vi "Begin.vi"() -> (0 "CameraDevRef 2":T1, 1 "CameraDevRef":T1)   [LabVIEW 2011]
doc: "Called before other user functions, this VI is expected to open initial I/O refnums, load in file data, and do all program initialization. Notice that the <B>error out</B> terminal is simply used for data flow. Wiring it to other structures or subVIs ensures that this VI runs first."
uses:
  <vilib>/Rock Robotics/WPI/Camera/WPI_CameraDevRef.ctl
  <vilib>/Rock Robotics/SystemInterfaces/DIO/FPGA_DIOPWMChannel.ctl
  <vilib>/Rock Robotics/WPI/Joystick/WPI_JoystickDeviceEnum.ctl
  <vilib>/Rock Robotics/SystemInterfaces/AI/FPGA_AIChannel.ctl
  <vilib>/Rock Robotics/SystemInterfaces/DIO/FPGA_DIORelayChannel.ctl
  <vilib>/Rock Robotics/SystemInterfaces/DIO/FPGA_DIOChannel.ctl
  <vilib>/Rock Robotics/SystemInterfaces/AI/FPGA_AIGyroChannel.ctl
  <vilib>/Rock Robotics/WPI/Relay/WPI_RelayDirection.ctl
  <vilib>/Rock Robotics/WPI/Encoder/WPI_EncoderType.ctl
  <vilib>/Rock Robotics/WPI/DriverStation/DriverStationLCD/WPI_DriverStationLCDLCDLine.ctl
  <vilib>/Rock Robotics/WPI/MotorControl/WPI_MotorControlOpen Victor.vi
  <vilib>/Rock Robotics/WPI/MotorControl/WPI_MotorControlOpen Jaguar.vi
  Robot Global Data.vi
  <vilib>/Utility/file.llb/Read From Spreadsheet File (DBL).vi
  <vilib>/Rock Robotics/WPI/Counter/WPI_CounterDigitalInputToDigitalSource.vi
  <vilib>/Rock Robotics/SystemInterfaces/Typedef/FPGA_TypedefDigitalModule.ctl
  <vilib>/Rock Robotics/SystemInterfaces/Typedef/FPGA_TypedefAnalogModule.ctl
panel:
  out "Path and file":string
  in  "Balls In Robot At Start":dbl=2.0
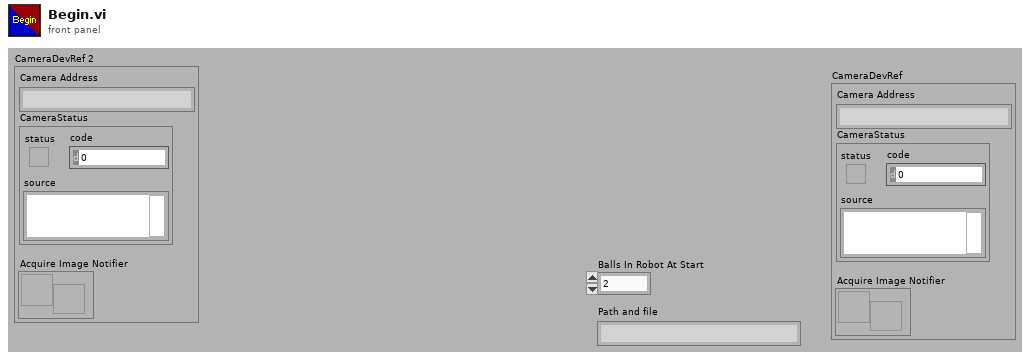
[diagram p1: front panel]
types:
  T1 = typedef "WPI_CameraDevRef.ctl" = cluster{"Camera Address":string, "CameraStatus":errorcluster, "Acquire Image Notifier":refnum<notifier>}
  T2 = typedef "WPI_DriverStationLCDLCDLine.ctl" = enum16{"Main - Line 1", "User - Line 2", "User - Line 3", "User - Line 4", "User - Line 5", "User - Line 6"}
  T3 = typedef "WPI_EncoderType.ctl" = enum16{"1x", "2x", "4x"}
  T4 = typedef "FPGA_DIOChannel.ctl" = enum8{"DIO 1", "DIO 2", "DIO 3", "DIO 4", "DIO 5", "DIO 6", "DIO 7", "DIO 8", "DIO 9", "DIO 10", "DIO 11", "DIO 12", "DIO 13", "DIO 14", "Invalid"}
  T5 = typedef "FPGA_DIORelayChannel.ctl" = enum8{"Relay 1", "Relay 2", "Relay 3", "Relay 4", "Relay 5", "Relay 6", "Relay 7", "Relay 8", "Invalid"}
  T6 = typedef "WPI_RelayDirection.ctl" = enum16{"Both directions", "Forward only", "Reverse only"}
  T7 = typedef "FPGA_AIGyroChannel.ctl" = enum8{"AI 1", "AI 2", "Invalid"}
  T8 = typedef "FPGA_DIOPWMChannel.ctl" = enum8{"PWM 1", "PWM 2", "PWM 3", "PWM 4", "PWM 5", "PWM 6", "PWM 7", "PWM 8", "PWM 9", "PWM 10", "Invalid"}
  T9 = typedef "FPGA_AIChannel.ctl" = enum8{"AI 1", "AI 2", "AI 3", "AI 4", "AI 5", "AI 6", "AI 7", "AI 8", "Invalid"}
  T10 = typedef "WPI_JoystickDeviceEnum.ctl" = enum16{"USB 1", "USB 2", "USB 3", "USB 4", "Kinect 1", "Kinect 2"}
  T11 = typedef "WPI_CameraImageSize.ctl" = enum16{"640x480", "320x240", "160x120"}
  T12 = cluster{"fps":i32, "compression":i32, "Image Size":T11}
  T13 = typedef "WPI_MotorControlDeviceRef.ctl" = cluster{"DeviceStatus":errorcluster, "Type":enum16{"PWM", "CAN"}, "PWM":cluster{"Digital Module":T14, "PWM Channel":T8, "DeadBand":T15}, "CAN":cluster{"Device Number":u8, "Control Mode":T16, "Semaphore":T17, "Max Vout":dbl}, "Invert":bool, "TransformRef":T18, "InvTransformRef":T18}
  T14 = typedef "FPGA_TypedefDigitalModule.ctl" = enum16{"Digital Module 1", "Digital Module 2"}
  T15 = typedef "WPI_PWMDeadband.ctl" = cluster{"Name":string, "maxPositivePwm":i32, "minPositivePwm":i32, "centerPwm":i32, "maxNegativePwm":i32, "minNegativePwm":i32, "angularRange":u16}
  T16 = typedef "WPI_CANJaguar_ControlMode.ctl" = enum8{"Percent VBus", "Current", "Speed", "Position", "Voltage"}
  T17 = typedef "Semaphore RefNum" = refnum<k1>
  T18 = typedef "WPI_PWMTransform_ConPane.ctl" = refnum<vi>
  T19 = typedef "WPI_ServoDeviceRef.ctl" = cluster{"DeviceStatus":errorcluster, "Digital Module":T14, "PWM Channel":T8, "DeadBand":T15}
  T20 = typedef "WPI_AnalogChannelDevRef.ctl" = cluster{"DevStatus":errorcluster, "Analog Module":T21, "Analog Channel":T9}
  T21 = typedef "FPGA_TypedefAnalogModule.ctl" = enum16{"Analog Module 1", "Analog Module 2"}
  T22 = typedef "WPI_CameraWhite Balance Values.ctl" = enum16{"Auto", "Fixed indoor", "Fixed outdoor 1", "Fixed outdoor 2", "Fixed fluorescent 1", "Fixed fluorescent 2", "Hold current"}
  T23 = typedef "WPI_JoystickDevRef.ctl" = cluster{"Device":T10}
  T24 = typedef "WPI_RelayDevRef.ctl" = cluster{"DevStatus":errorcluster, "Relay Channel":T5, "Digital Module":T14, "Relay Direction":T6}
  T25 = typedef "WPI_CameraExposure Values.ctl" = enum16{"Auto", "Flicker-free 50 Hz", "Flicker-free 60 Hz", "Hold current"}
  T26 = typedef "WPI_DigitalInputDevRef.ctl" = cluster{"DevStatus":errorcluster, "DIO Channel":T4, "Digital Module":T14}
  T27 = typedef "FPGA_CounterEncoderSourceConvertionLVSourceType.ctl" = cluster{"DevStatus":errorcluster, "AnalogTriggerMode?":bool, "DigitalMode":cluster{"Digital Module":T14, "DIO Channel":T28}, "AnalogTriggerMode":cluster{"AnalogTriggerIndex":T29, "OutputType":T30}}
  T28 = typedef "FPGA_DIODigitalSourceChannel.ctl" = enum8{"DIO 1", "DIO 2", "DIO 3", "DIO 4", "DIO 5", "DIO 6", "DIO 7", "DIO 8", "DIO 9", "DIO 10", "DIO 11", "DIO 12", "DIO 13", "DIO 14", "Disabled"}
  T29 = typedef "FPGA_AnalogTriggerIndex.ctl" = enum8{"Trig 0", "Trig 1", "Trig 2", "Trig 3", "Trig 4", "Trig 5", "Trig 6", "Trig 7", "Invalid"}
  T30 = typedef "FPGA_AnalogTriggerOutType.ctl" = enum16{"InWindow", "TriggerState", "Rising", "Falling"}
  T31 = typedef "WPI_EncoderDevRef.ctl" = cluster{"DevStatus":errorcluster, "EncoderIndex":T32, "CounterIndex":T33, "DistancePerCount":dbl, "Decoding Type":T3}
  T32 = typedef "FPGA_EncoderIdx.ctl" = enum8{"Enc 0", "Enc 1", "Enc 2", "Enc 3", "Invalid"}
  T33 = typedef "FPGA_CounterCtrSystemIndex.ctl" = enum8{"Ctr 0", "Ctr 1", "Ctr 2", "Ctr 3", "Ctr 4", "Ctr 5", "Ctr 6", "Ctr 7", "Invalid"}
  T34 = typedef "WPI_GyroDevRef.ctl" = cluster{"DevStatus":errorcluster, "Analog Module":T21, "Analog Channel":T9, "Offset":dbl, "Gain (VoltsPerDegree/Second)":dbl}
  T35 = typedef "WPI_UltrasonicDeviceRef.ctl" = cluster{"DevStatus":errorcluster, "Ping Digital Module":T14, "Echo Digital Module":T14, "Ping Channel":T4, "Echo Channel":T4, "CntIndex":T33}
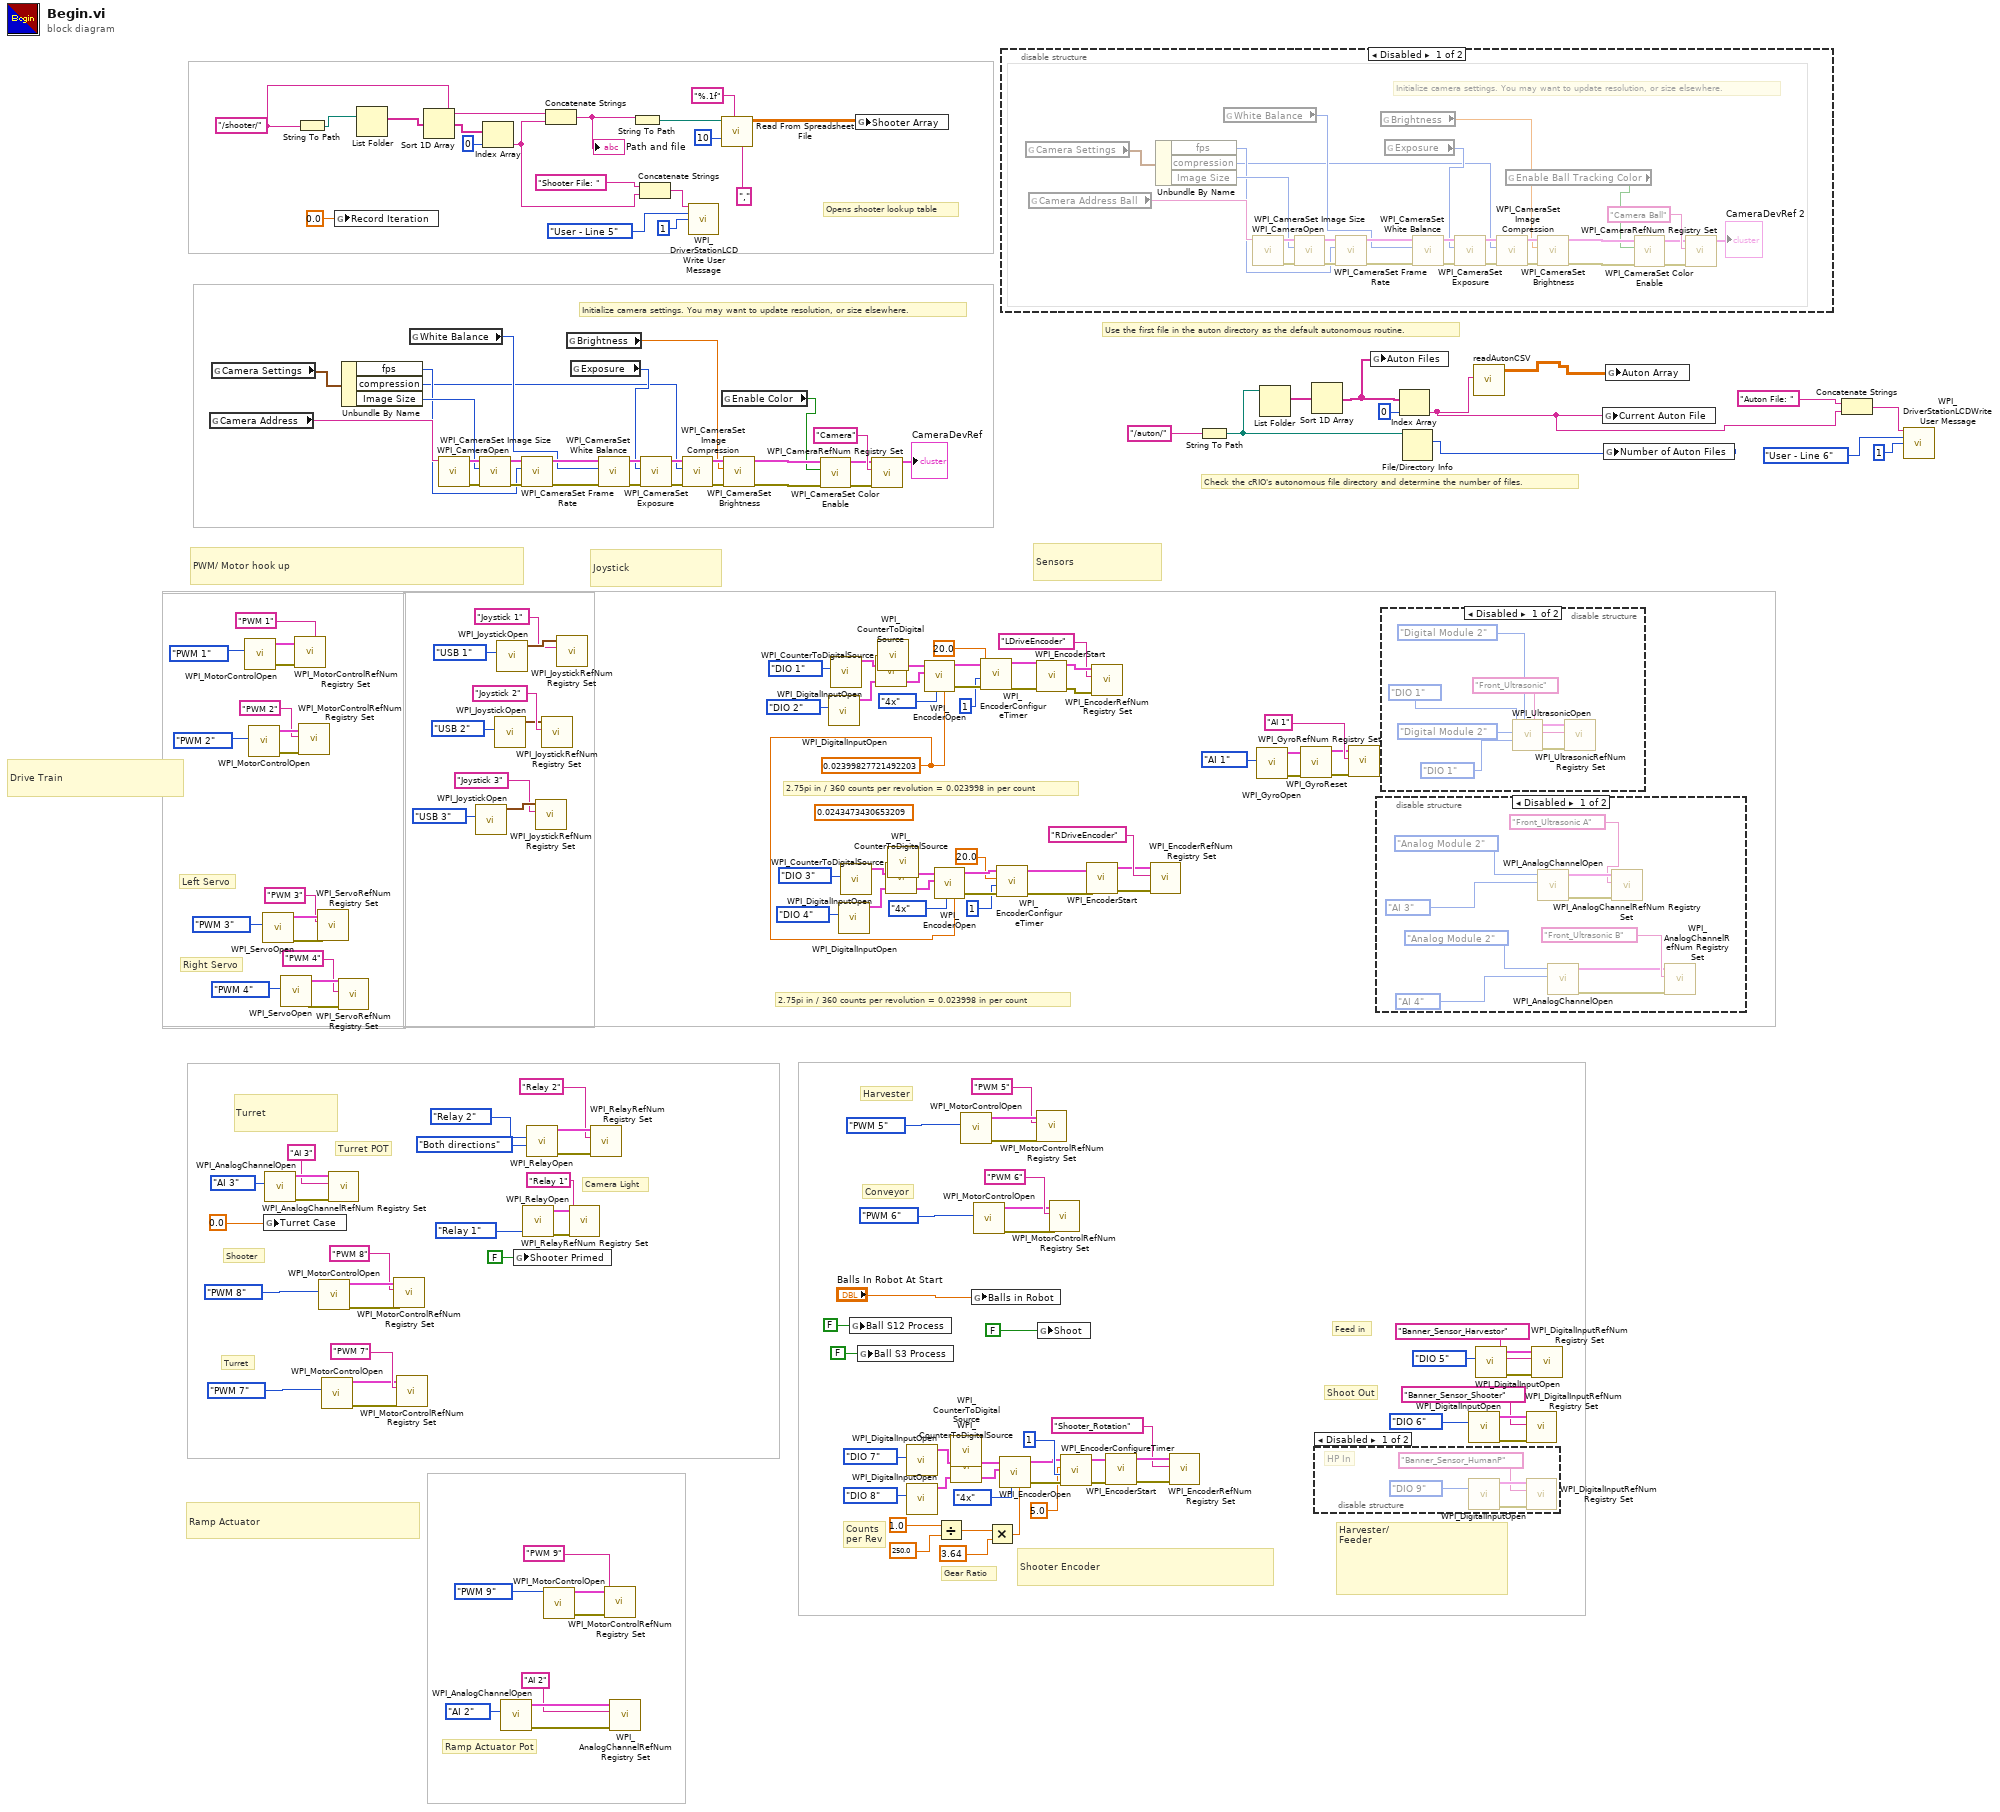
[diagram p0: block diagram]
diagram:
  (unwired) 0.0243473430653209 ("DistancePerCount")
  w32 = 0.02399827721492203 ("DistancePerCount")
  w80 = "/shooter/" ("string")
  # "Shooter Encoder"
  # "Counts\nper Rev"
  # "Gear Ratio"
  # "Check the cRIO's autonomous file directory and determine the number of files."
  # "Use the first file in the auton directory as the default autonomous routine."
  # "2.75pi in / 360 counts per revolution = 0.023998 in per count"
  # "2.75pi in / 360 counts per revolution = 0.023998 in per count"
  # "Opens shooter lookup table"
  # "Shoot Out"
  # "Feed in"
  # "Harvester"
  # "Conveyor"
  # "Shooter"
  # "Initialize camera settings. You may want to update resolution, or size elsewhere."
  # "Camera Light"
  # "Ramp Actuator Pot"
  # "Turret POT"
  # "Turret"
  # "Right Servo"
  # "Left Servo"
  # "Harvester/\nFeeder"
  # "Turret"
  # "Ramp Actuator"
  # "Drive Train"
  # "Sensors"
  # "Joystick"
  # "PWM/ Motor hook up"
  n1 = global read "Robot Global Data.vi" "Camera Address"() -> (w133:string)
  n2 = global read "Robot Global Data.vi" "Camera Settings"() -> (w132:T12)
  n3 = call-poly <vilib>:"WPI_MotorControlOpen.vi"("PWM Channel"=FPGA_DIOPWMChannel."PWM 1") -> ("error out"=w173:errorcluster, "MotorControlDeviceRef"=w175:T13)  [unwired: 9 in]
  n4 = call-poly <vilib>:"WPI_MotorControlOpen.vi"("PWM Channel"=FPGA_DIOPWMChannel."PWM 2") -> ("error out"=w171:errorcluster, "MotorControlDeviceRef"=w169:T13)  [unwired: 9 in]
  n5 = call <vilib>:"WPI_ServoOpen.vi"("PWM Channel"=FPGA_DIOPWMChannel."PWM 3") -> ("error out"=w186:errorcluster, "ServoDeviceRef"=w191:T19)  [unwired: 9 in]
  n6 = global write "Robot Global Data.vi" "Turret Case"(0.0 ("Return To Home Case")) -> ()
  n7 = call <vilib>:"WPI_AnalogChannelOpen.vi"("Analog Channel"=FPGA_AIChannel."AI 3") -> ("error out"=w162:errorcluster, "AIDeviceRef"=w163:T20)  [unwired: 9 in]
  n8 = call <vilib>:"WPI_ServoOpen.vi"("PWM Channel"=FPGA_DIOPWMChannel."PWM 4") -> ("error out"=w185:errorcluster, "ServoDeviceRef"=w189:T19)  [unwired: 9 in]
  n9 = call <vilib>:"WPI_MotorControlRefNum Registry Set.vi"("error in (no error)"=w173, "refnum name"="PWM 1", "MotorControlDevRef"=w175) -> ()  [unwired: 7 in, 2 out]
  n10 = String To Path(string=w80) -> (path=w89:path)
  n11 = call <vilib>:"WPI_MotorControlRefNum Registry Set.vi"("error in (no error)"=w171, "refnum name"="PWM 2", "MotorControlDevRef"=w169) -> ()  [unwired: 7 in, 2 out]
  n12 = call <vilib>:"WPI_ServoRefNum Registry Set.vi"("error in (no error)"=w186, "refnum name"="PWM 3", "ServoDeviceRef"=w191) -> ()  [unwired: 7 in, 2 out]
  n13 = call-poly <vilib>:"WPI_MotorControlOpen.vi"("PWM Channel"=FPGA_DIOPWMChannel."PWM 8") -> ("error out"=w116:errorcluster, "MotorControlDeviceRef"=w118:T13)  [unwired: 9 in]
  n14 = call-poly <vilib>:"WPI_MotorControlOpen.vi"("PWM Channel"=FPGA_DIOPWMChannel."PWM 7") -> ("error out"=w167:errorcluster, "MotorControlDeviceRef"=w165:T13)  [unwired: 9 in]
  n15 = call <vilib>:"WPI_AnalogChannelRefNum Registry Set.vi"("error in (no error)"=w162, "refnum name"="AI 3", "AIDeviceRef"=w163) -> ()  [unwired: 7 in, 2 out]
  n16 = global write "Robot Global Data.vi" "Record Iteration"(0.0 ("Record Iteration")) -> ()
  n17 = call <vilib>:"WPI_ServoRefNum Registry Set.vi"("error in (no error)"=w185, "refnum name"="PWM 4", "ServoDeviceRef"=w189) -> ()  [unwired: 7 in, 2 out]
  n18 = Unbundle By Name(w132) -> ("fps"=w130:i32, "compression"=w127:i32, "Image Size"=w131:T11)
  n19 = List Folder(path=w89) -> (filenames=w88:string[])  [unwired: 1 in, 5 out]
  n20 = call <vilib>:"WPI_MotorControlRefNum Registry Set.vi"("error in (no error)"=w116, "refnum name"="PWM 8", "MotorControlDevRef"=w118) -> ()  [unwired: 7 in, 2 out]
  n21 = call <vilib>:"WPI_MotorControlRefNum Registry Set.vi"("error in (no error)"=w167, "refnum name"="PWM 7", "MotorControlDevRef"=w165) -> ()  [unwired: 7 in, 2 out]
  n22 = global read "Robot Global Data.vi" "White Balance"() -> (w129:T22)
  n23 = Sort 1D Array(array=w88) -> (sorted array=w87:string[])
  n24 = call <vilib>:"WPI_CameraOpen.vi"("Camera Address"=w133) -> ("error out"=w139:errorcluster, "CameraDevRef"=w140:T1)  [unwired: 1 in, 8 out]
  n25 = call <vilib>:"WPI_JoystickOpen.vi"("JoystickDevice"=WPI_JoystickDeviceEnum."USB 3") -> ("JoystickDevRef"=w178:T23)  [unwired: 10 in]
  n26 = call <vilib>:"WPI_CameraSet Image Size.vi"("error in (no error)"=w139, "Image Size"=w131, "CameraDevRef"=w140) -> ("error out"=w138:errorcluster, "CameraDevRef Out"=w141:T1)  [unwired: 7 out]
  n27 = Index Array(array=w87, index=0) -> (element=w6:string)
  n28 = call <vilib>:"WPI_JoystickOpen.vi"("JoystickDevice"=WPI_JoystickDeviceEnum."USB 2") -> ("JoystickDevRef"=w181:T23)  [unwired: 10 in]
  n29 = call <vilib>:"WPI_JoystickOpen.vi"("JoystickDevice"=WPI_JoystickDeviceEnum."USB 1") -> ("JoystickDevRef"=w184:T23)  [unwired: 10 in]
  n30 = call <vilib>:"WPI_AnalogChannelOpen.vi"("Analog Channel"=FPGA_AIChannel."AI 2") -> ("error out"=w157:errorcluster, "AIDeviceRef"=w158:T20)  [unwired: 9 in]
  n31 = global write "Robot Global Data.vi" "Shooter Primed"(FALSE ("Ball S3 Process")) -> ()
  n32 = call <vilib>:"WPI_CameraSet Frame Rate.vi"("error in (no error)"=w138, "Frame Rate (fps)"=w130, "CameraDevRef"=w141) -> ("error out"=w137:errorcluster, "CameraDevRef Out"=w143:T1)  [unwired: 7 out]
  n33 = call <vilib>:"WPI_RelayOpen.vi"("Relay Channel"=FPGA_DIORelayChannel."Relay 1") -> ("error out"=w150:errorcluster, "RelayDevRef"=w149:T24)  [unwired: 9 in]
  n34 = call <vilib>:"WPI_RelayOpen.vi"("Relay Direction"=WPI_RelayDirection."Both directions", "Relay Channel"=FPGA_DIORelayChannel."Relay 2") -> ("error out"=w75:errorcluster, "RelayDevRef"=w76:T24)  [unwired: 8 in]
  n35 = call <vilib>:"WPI_JoystickRefNum Registry Set.vi"("refnum name"="Joystick 3", "JoystickDevRef"=w178) -> ()  [unwired: 8 in, 2 out]
  n36 = call <vilib>:"WPI_JoystickRefNum Registry Set.vi"("refnum name"="Joystick 2", "JoystickDevRef"=w181) -> ()  [unwired: 8 in, 2 out]
  n37 = call-poly <vilib>:"WPI_MotorControlOpen.vi"("PWM Channel"=FPGA_DIOPWMChannel."PWM 9") -> ("error out"=w153:errorcluster, "MotorControlDeviceRef"=w154:T13)  [unwired: 9 in]
  n38 = Concatenate Strings(w80, w6) -> (w82:string)
  "Path and file" <- w82
  n39 = call <vilib>:"WPI_JoystickRefNum Registry Set.vi"("refnum name"="Joystick 1", "JoystickDevRef"=w184) -> ()  [unwired: 8 in, 2 out]
  n40 = global read "Robot Global Data.vi" "Brightness"() -> (w126:dbl)
  n41 = call <vilib>:"WPI_RelayRefNum Registry Set.vi"("error in (no error)"=w150, "refnum name"="Relay 1", "RelayDevRef"=w149) -> ()  [unwired: 7 in, 2 out]
  n42 = global read "Robot Global Data.vi" "Exposure"() -> (w128:T25)
  n43 = call <vilib>:"WPI_RelayRefNum Registry Set.vi"("error in (no error)"=w75, "refnum name"="Relay 2", "RelayDevRef"=w76) -> ()  [unwired: 7 in, 2 out]
  n44 = call <vilib>:"WPI_CameraSet White Balance.vi"("error in (no error)"=w137, "White Balance"=w129, "CameraDevRef"=w143) -> ("error out"=w136:errorcluster, "CameraDevRef Out"=w142:T1)  [unwired: 7 out]
  n45 = call <vilib>:"WPI_MotorControlRefNum Registry Set.vi"("error in (no error)"=w153, "refnum name"="PWM 9", "MotorControlDevRef"=w154) -> ()  [unwired: 7 in, 2 out]
  n46 = call <vilib>:"WPI_AnalogChannelRefNum Registry Set.vi"("error in (no error)"=w157, "refnum name"="AI 2", "AIDeviceRef"=w158) -> ()  [unwired: 7 in, 2 out]
  n47 = String To Path(string=w82) -> (path=w81:path)
  n48 = Concatenate Strings("Shooter File: ", w6) -> (w4:string)
  n49 = call <vilib>:"WPI_CameraSet Exposure.vi"("error in (no error)"=w136, "Exposure"=w128, "CameraDevRef"=w142) -> ("error out"=w135:errorcluster, "CameraDevRef Out"=w145:T1)  [unwired: 7 out]
  n50 = call <vilib>:"WPI_CameraSet Image Compression.vi"("error in (no error)"=w135, "Compression"=w127, "CameraDevRef"=w145) -> ("error out"=w134:errorcluster, "CameraDevRef Out"=w144:T1)  [unwired: 7 out]
  n51 = call <vilib>:"WPI_DriverStationLCDWrite User Message.vi"("line text"=w4, "line"=WPI_DriverStationLCDLCDLine."User - Line 5", "starting column"=i8 1) -> ()  [unwired: 2 in, 11 out]
  n52 = call-poly <vilib>:"Read From Spreadsheet File.vi"("delimiter (\\t)"="," ("delimiter (\\t)"), "format (%.3f)"="%.1f", "number of rows (all:-1)"=10, "file path (dialog if empty)"=w81) -> ("all rows"=w79:dbl[][])  [unwired: 1 in, 6 out]
  n53 = global read "Robot Global Data.vi" "Enable Color"() -> (w121:bool)
  n54 = call <vilib>:"WPI_CameraSet Brightness.vi"("error in (no error)"=w134, "Brightness"=w126, "CameraDevRef"=w144) -> ("error out"=w124:errorcluster, "CameraDevRef Out"=w125:T1)  [unwired: 7 out]
  n55 = call <vilib>:"WPI_CameraSet Color Enable.vi"("error in (no error)"=w124, "Color Enabled"=w121, "CameraDevRef"=w125) -> ("error out"=w122:errorcluster, "CameraDevRef Out"=w123:T1)  [unwired: 7 in]
  n56 = call <vilib>:"WPI_DigitalInputOpen.vi"("DIO Channel"=FPGA_DIOChannel."DIO 2") -> ("DigitalInputDevRef"=w67:T26)  [unwired: 9 in, 1 out]
  n57 = call <vilib>:"WPI_DigitalInputOpen.vi"("DIO Channel"=FPGA_DIOChannel."DIO 1") -> ("DigitalInputDevRef"=w64:T26)  [unwired: 9 in, 1 out]
  n58 = call <vilib>:"WPI_DigitalInputOpen.vi"("DIO Channel"=FPGA_DIOChannel."DIO 4") -> ("DigitalInputDevRef"=w58:T26)  [unwired: 9 in, 1 out]
  n59 = call <vilib>:"WPI_DigitalInputOpen.vi"("DIO Channel"=FPGA_DIOChannel."DIO 3") -> ("DigitalInputDevRef"=w61:T26)  [unwired: 9 in, 1 out]
  n60 = global write "Robot Global Data.vi" "Ball S12 Process"(FALSE ("Ball S12 Process")) -> ()
  n61 = global write "Robot Global Data.vi" "Shooter Array"(w79) -> ()
  n62 = global write "Robot Global Data.vi" "Ball S3 Process"(FALSE ("Ball S3 Process")) -> ()
  n63 = call <vilib>:"WPI_CameraRefNum Registry Set.vi"("error in (no error)"=w122, "refnum name"="Camera", "CameraDevRef"=w123) -> ("CameraDevRef"=→"CameraDevRef":T1)  [unwired: 8 out]
  n64 = call-poly <vilib>:"WPI_CounterToDigitalSource.vi"("DigitalInputDevRef"=w67) -> ("Digital Source"=w68:T27)  [unwired: 6 in]
  n65 = call-poly <vilib>:"WPI_CounterToDigitalSource.vi"("DigitalInputDevRef"=w64) -> ("Digital Source"=w63:T27)  [unwired: 6 in]
  n66 = call-poly <vilib>:"WPI_CounterToDigitalSource.vi"("DigitalInputDevRef"=w58) -> ("Digital Source"=w57:T27)  [unwired: 6 in]
  n67 = call-poly <vilib>:"WPI_CounterToDigitalSource.vi"("DigitalInputDevRef"=w61) -> ("Digital Source"=w62:T27)  [unwired: 6 in]
  n68 = call <vilib>:"WPI_DigitalInputOpen.vi"("DIO Channel"=FPGA_DIOChannel."DIO 7") -> ("DigitalInputDevRef"=w16:T26)  [unwired: 9 in, 1 out]
  n69 = call <vilib>:"WPI_DigitalInputOpen.vi"("DIO Channel"=FPGA_DIOChannel."DIO 8") -> ("DigitalInputDevRef"=w19:T26)  [unwired: 9 in, 1 out]
  n70 = call <vilib>:"WPI_EncoderOpen.vi"("DistancePerCount"=w32, "Decoding Type"=WPI_EncoderType."4x", "BSource"=w68, "ASource"=w63) -> ("error out"=w36:errorcluster, "EncoderDevRef"=w39:T31)  [unwired: 6 in]
  n71 = call <vilib>:"WPI_EncoderOpen.vi"("DistancePerCount"=w32, "Decoding Type"=WPI_EncoderType."4x", "BSource"=w57, "ASource"=w62) -> ("error out"=w54:errorcluster, "EncoderDevRef"=w53:T31)  [unwired: 6 in]
  n72 = Divide(x=1.0, y=250.0) -> (x/y=w13:dbl)
  n73 = call-poly <vilib>:"WPI_CounterToDigitalSource.vi"("DigitalInputDevRef"=w16) -> ("Digital Source"=w15:T27)  [unwired: 6 in]
  n74 = call-poly <vilib>:"WPI_CounterToDigitalSource.vi"("DigitalInputDevRef"=w19) -> ("Digital Source"=w20:T27)  [unwired: 6 in]
  n75 = call-poly <vilib>:"WPI_MotorControlOpen.vi"("PWM Channel"=FPGA_DIOPWMChannel."PWM 5") -> ("error out"=w112:errorcluster, "MotorControlDeviceRef"=w114:T13)  [unwired: 9 in]
  n76 = global write "Robot Global Data.vi" "Balls in Robot"("Balls In Robot At Start") -> ()
  n77 = call-poly <vilib>:"WPI_MotorControlOpen.vi"("PWM Channel"=FPGA_DIOPWMChannel."PWM 6") -> ("error out"=w111:errorcluster, "MotorControlDeviceRef"=w109:T13)  [unwired: 9 in]
  n78 = call <vilib>:"WPI_EncoderConfigureTimer.vi"("error in (no error)"=w36, "Number Samples to Average"=u8 1, "Minimum Rate"=20.0, "EncoderDevRef"=w39) -> ("error out"=w37:errorcluster, "EncoderDevRef"=w38:T31)  [unwired: 6 in]
  n79 = Multiply(x=w13, y=3.64) -> (x*y=w11:dbl)
  n80 = call <vilib>:"WPI_EncoderConfigureTimer.vi"("error in (no error)"=w54, "Number Samples to Average"=u8 1, "Minimum Rate"=20.0, "EncoderDevRef"=w53) -> ("error out"=w50:errorcluster, "EncoderDevRef"=w51:T31)  [unwired: 6 in]
  n81 = call <vilib>:"WPI_EncoderOpen.vi"("DistancePerCount"=w11, "Decoding Type"=WPI_EncoderType."4x", "BSource"=w20, "ASource"=w15) -> ("error out"=w23:errorcluster, "EncoderDevRef"=w24:T31)  [unwired: 6 in]
  n82 = disable-structure shown="Disabled" {
    frame Disabled {
      # "Initialize camera settings. You may want to update resolution, or size elsewhere."
      n83 = global read "Robot Global Data.vi" "Camera Settings"() -> (w205:T12)
      n84 = global read "Robot Global Data.vi" "Camera Address Ball"() -> (w206:string)
      n85 = Unbundle By Name(w205) -> ("fps"=w203:i32, "compression"=w200:i32, "Image Size"=w204:T11)
      n86 = global read "Robot Global Data.vi" "White Balance"() -> (w202:T22)
      n87 = call <vilib>:"WPI_CameraOpen.vi"("Camera Address"=w206) -> ("error out"=w212:errorcluster, "CameraDevRef"=w213:T1)  [unwired: 1 in, 8 out]
      n88 = call <vilib>:"WPI_CameraSet Image Size.vi"("error in (no error)"=w212, "Image Size"=w204, "CameraDevRef"=w213) -> ("error out"=w211:errorcluster, "CameraDevRef Out"=w214:T1)  [unwired: 7 out]
      n89 = call <vilib>:"WPI_CameraSet Frame Rate.vi"("error in (no error)"=w211, "Frame Rate (fps)"=w203, "CameraDevRef"=w214) -> ("error out"=w210:errorcluster, "CameraDevRef Out"=w216:T1)  [unwired: 7 out]
      n90 = global read "Robot Global Data.vi" "Brightness"() -> (w199:dbl)
      n91 = global read "Robot Global Data.vi" "Exposure"() -> (w201:T25)
      n92 = call <vilib>:"WPI_CameraSet White Balance.vi"("error in (no error)"=w210, "White Balance"=w202, "CameraDevRef"=w216) -> ("error out"=w209:errorcluster, "CameraDevRef Out"=w215:T1)  [unwired: 7 out]
      n93 = call <vilib>:"WPI_CameraSet Exposure.vi"("error in (no error)"=w209, "Exposure"=w201, "CameraDevRef"=w215) -> ("error out"=w208:errorcluster, "CameraDevRef Out"=w218:T1)  [unwired: 7 out]
      n94 = call <vilib>:"WPI_CameraSet Image Compression.vi"("error in (no error)"=w208, "Compression"=w200, "CameraDevRef"=w218) -> ("error out"=w207:errorcluster, "CameraDevRef Out"=w217:T1)  [unwired: 7 out]
      n95 = global read "Robot Global Data.vi" "Enable Ball Tracking Color"() -> (w194:bool)
      n96 = call <vilib>:"WPI_CameraSet Brightness.vi"("error in (no error)"=w207, "Brightness"=w199, "CameraDevRef"=w217) -> ("error out"=w197:errorcluster, "CameraDevRef Out"=w198:T1)  [unwired: 7 out]
      n97 = call <vilib>:"WPI_CameraSet Color Enable.vi"("error in (no error)"=w197, "Color Enabled"=w194, "CameraDevRef"=w198) -> ("error out"=w195:errorcluster, "CameraDevRef Out"=w196:T1)  [unwired: 7 in]
      n98 = call <vilib>:"WPI_CameraRefNum Registry Set.vi"("error in (no error)"=w195, "refnum name"="Camera Ball", "CameraDevRef"=w196) -> ("CameraDevRef"=→"CameraDevRef 2":T1)  [unwired: 8 out]
    }
    frame Enabled {
    }
  }
  n99 = call <vilib>:"WPI_EncoderStart.vi"("error in (no error)"=w37, "EncoderDevRef"=w38) -> ("error out"=w71:errorcluster, "EncoderDevRef"=w70:T31)  [unwired: 8 in]
  n100 = call <vilib>:"WPI_MotorControlRefNum Registry Set.vi"("error in (no error)"=w112, "refnum name"="PWM 5", "MotorControlDevRef"=w114) -> ()  [unwired: 7 in, 2 out]
  n101 = global write "Robot Global Data.vi" "Shoot"(FALSE ("Ball S12 Process")) -> ()
  n102 = call <vilib>:"WPI_MotorControlRefNum Registry Set.vi"("error in (no error)"=w111, "refnum name"="PWM 6", "MotorControlDevRef"=w109) -> ()  [unwired: 7 in, 2 out]
  n103 = call <vilib>:"WPI_EncoderConfigureTimer.vi"("error in (no error)"=w23, "Number Samples to Average"=u8 1, "Minimum Rate"=5.0, "EncoderDevRef"=w24) -> ("error out"=w27:errorcluster, "EncoderDevRef"=w26:T31)  [unwired: 6 in]
  n104 = call <vilib>:"WPI_EncoderStart.vi"("error in (no error)"=w50, "EncoderDevRef"=w51) -> ("error out"=w48:errorcluster, "EncoderDevRef"=w49:T31)  [unwired: 8 in]
  n105 = call <vilib>:"WPI_EncoderRefNum Registry Set.vi"("error in (no error)"=w71, "refnum name"="LDriveEncoder", "EncoderDevRef"=w70) -> ()  [unwired: 7 in, 2 out]
  n106 = call <vilib>:"WPI_EncoderStart.vi"("error in (no error)"=w27, "EncoderDevRef"=w26) -> ("error out"=w29:errorcluster, "EncoderDevRef"=w28:T31)  [unwired: 8 in]
  n107 = call <vilib>:"WPI_EncoderRefNum Registry Set.vi"("error in (no error)"=w48, "refnum name"="RDriveEncoder", "EncoderDevRef"=w49) -> ()  [unwired: 7 in, 2 out]
  n108 = call <vilib>:"WPI_EncoderRefNum Registry Set.vi"("error in (no error)"=w29, "refnum name"="Shooter_Rotation", "EncoderDevRef"=w28) -> ()  [unwired: 7 in, 2 out]
  n109 = String To Path(string="/auton/") -> (path=w44:path)
  n110 = call <vilib>:"WPI_GyroOpen.vi"("Analog Channel"=FPGA_AIGyroChannel."AI 1") -> ("error out"=w92:errorcluster, "GyroDevRef"=w93:T34)  [unwired: 8 in, 1 out]
  n111 = List Folder(path=w44) -> (filenames=w43:string[])  [unwired: 1 in, 5 out]
  n112 = call <vilib>:"WPI_GyroReset.vi"("error in (no error)"=w92, "GyroDevRef"=w93) -> ("error out"=w91:errorcluster, "GyroDevRef"=w90:T34)  [unwired: 8 in]
  n113 = Sort 1D Array(array=w43) -> (sorted array=w41:string[])
  n114 = disable-structure shown="Disabled" {
    frame Disabled {
      # "HP In"
      n115 = call <vilib>:"WPI_DigitalInputOpen.vi"("DIO Channel"=FPGA_DIOChannel."DIO 9") -> ("error out"=w222:errorcluster, "DigitalInputDevRef"=w221:T26)  [unwired: 9 in]
      n116 = call <vilib>:"WPI_DigitalInputRefNum Registry Set.vi"("error in (no error)"=w222, "refnum name"="Banner_Sensor_HumanP", "DigitalInputDevRef"=w221) -> ()  [unwired: 7 in, 2 out]
    }
    frame Enabled {
    }
  }
  n117 = call <vilib>:"WPI_GyroRefNum Registry Set.vi"("error in (no error)"=w91, "refnum name"="AI 1", "GyroDevRef"=w90) -> ()  [unwired: 7 in, 2 out]
  n118 = global write "Robot Global Data.vi" "Auton Files"(w41) -> ()
  n119 = disable-structure shown="Disabled" {
    frame Disabled {
      n120 = call <vilib>:"WPI_AnalogChannelOpen.vi"("Analog Channel"=FPGA_AIChannel."AI 3", "Analog Module (Module 1)"=FPGA_TypedefAnalogModule."Analog Module 2") -> ("error out"=w229:errorcluster, "AIDeviceRef"=w228:T20)  [unwired: 8 in]
      n121 = call <vilib>:"WPI_AnalogChannelOpen.vi"("Analog Channel"=FPGA_AIChannel."AI 4", "Analog Module (Module 1)"=FPGA_TypedefAnalogModule."Analog Module 2") -> ("error out"=w224:errorcluster, "AIDeviceRef"=w225:T20)  [unwired: 8 in]
      n122 = call <vilib>:"WPI_AnalogChannelRefNum Registry Set.vi"("error in (no error)"=w229, "refnum name"="Front_Ultrasonic A", "AIDeviceRef"=w228) -> ()  [unwired: 7 in, 2 out]
      n123 = call <vilib>:"WPI_AnalogChannelRefNum Registry Set.vi"("error in (no error)"=w224, "refnum name"="Front_Ultrasonic B", "AIDeviceRef"=w225) -> ()  [unwired: 7 in, 2 out]
    }
    frame Enabled {
    }
  }
  n124 = disable-structure shown="Disabled" {
    frame Disabled {
      n125 = call <vilib>:"WPI_UltrasonicOpen.vi"("Ping Digital Module (Module 1)"=FPGA_TypedefDigitalModule."Digital Module 2", "Echo DIO Channel"=FPGA_DIOChannel."DIO 1", "Echo Digital Module (Module 1)"=FPGA_TypedefDigitalModule."Digital Module 2", "Ping DIO Channel"=FPGA_DIOChannel."DIO 1") -> ("error out"=w240:errorcluster, "UltrasonicDevRef"=w239:T35)  [unwired: 6 in]
      n126 = call <vilib>:"WPI_UltrasonicRefNum Registry Set.vi"("error in (no error)"=w240, "refnum name"="Front_Ultrasonic", "UltrasonicDevRef"=w239) -> ()  [unwired: 7 in, 2 out]
    }
    frame Enabled {
    }
  }
  n127 = Index Array(array=w41, index=0) -> (element=w2:string)
  n128 = File/Directory Info(path=w44) -> (size=w46:i64)  [unwired: 1 in, 6 out]
  n129 = call <vilib>:"WPI_DigitalInputOpen.vi"("DIO Channel"=FPGA_DIOChannel."DIO 6") -> ("error out"=w102:errorcluster, "DigitalInputDevRef"=w101:T26)  [unwired: 9 in]
  n130 = call "readAutonCSV.vi"("AutonFile"=w2) -> ("AutonArray"=w40:dbl[][])  [unwired: 7 in]
  n131 = call <vilib>:"WPI_DigitalInputOpen.vi"("DIO Channel"=FPGA_DIOChannel."DIO 5") -> ("error out"=w105:errorcluster, "DigitalInputDevRef"=w104:T26)  [unwired: 9 in]
  n132 = call <vilib>:"WPI_DigitalInputRefNum Registry Set.vi"("error in (no error)"=w102, "refnum name"="Banner_Sensor_Shooter", "DigitalInputDevRef"=w101) -> ()  [unwired: 7 in, 2 out]
  n133 = call <vilib>:"WPI_DigitalInputRefNum Registry Set.vi"("error in (no error)"=w105, "refnum name"="Banner_Sensor_Harvestor", "DigitalInputDevRef"=w104) -> ()  [unwired: 7 in, 2 out]
  n134 = global write "Robot Global Data.vi" "Current Auton File"(w2) -> ()
  n135 = global write "Robot Global Data.vi" "Number of Auton Files"(w46) -> ()
  n136 = global write "Robot Global Data.vi" "Auton Array"(w40) -> ()
  n137 = Concatenate Strings("Auton File: ", w2) -> (w1:string)
  n138 = call <vilib>:"WPI_DriverStationLCDWrite User Message.vi"("line text"=w1, "line"=WPI_DriverStationLCDLCDLine."User - Line 6", "starting column"=i8 1) -> ()  [unwired: 2 in, 11 out]
